vi "Write Due Dates.vi"(8 "error in (no error)":errorcluster, 10 "Due Dates":u16[](array[numeric]), 11 "OSSP_Problem in":refnum<class "OSSP_Problem.lvclass">) -> (0 "error out":errorcluster, 3 "OSSP_Problem out":refnum<class "OSSP_Problem.lvclass">)   [LabVIEW 2013, in "OSSP_Problem.lvclass"]
uses:
  OSSP_Problem.lvclass
  OSSP_Problem.lvclass/OSSP_Problem.ctl
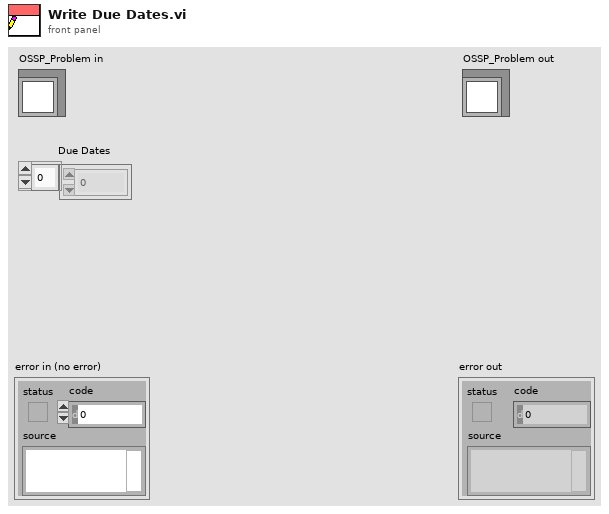
[diagram p1: front panel]
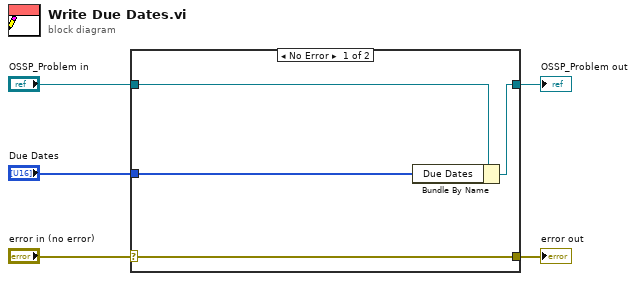
[diagram p0: block diagram]
diagram:
  n1 = case shown="No Error" "error in (no error)" {
    selector: "error in (no error)" -> [w9 w10]
    tunnel: [w9 w10] -> w4
    tunnel: [w7 w11] -> w2
    tunnel: "OSSP_Problem in" -> [w8 w11]
    tunnel: "Due Dates" -> [w6 _]
    frame No Error {
      n2 = Bundle By Name(cluster=w8, "Due Dates"=w6) -> (w7:refnum<class "OSSP_Problem.lvclass">)
    }
    frame Error {
    }
  }
  "error out" <- w4
  "OSSP_Problem out" <- w2
